vi "Configure VIs for Execution.vi"   [LabVIEW 2016, in "Memory.lvlib"]
uses:
  Memory.lvlib
types:
  T1 = enum32{"invalid VI type", "Standard VI", "Control VI", "Global VI", "Polymorphic VI", "Configuration VI", "SubSystem", "Facade VI", "Method VI", "Statechart Diagram VI"}
  T2 = enum16{"Share clones between instances", "Preallocate clone for each instance"}
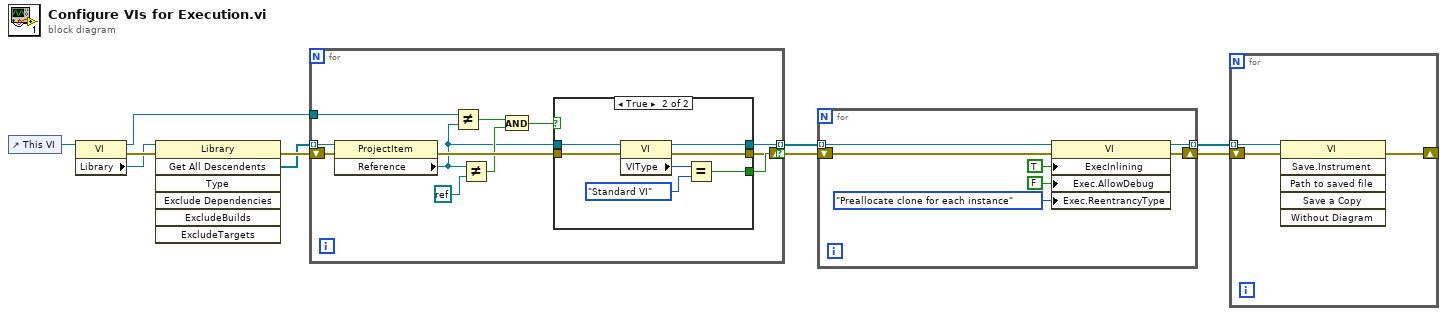
[diagram p0: block diagram]
diagram:
  n1 = control-ref of="This VI"() -> (w10:refnum<vi>)
  n2 = property class="VI"(reference=w10) -> (reference out=w8:refnum<vi>, error out=w3:errorcluster, "Library"=w1:refnum<vi>)  [unwired: 1 in]
  n3 = invoke class="Library" method="Get All Descendents"(reference=w1, error in=w3) -> (error out=w4:errorcluster, "All Descendents"=w2:refnum<vi>[])  [unwired: 5 in, 5 out]
  n4 = for {
    tunnel: w2 -> [w22] mode=indexing
    tunnel: [w21] -> w9 mode=indexing if=w20
    tunnel: w8 -> [w18]
    shift-right: [w16] -> w7
    shift-left: w4 -> [w15]
    n5 = property class="ProjectItem"(reference=w22, error in=w15) -> (error out=w14:errorcluster, "Reference"=w11:refnum<vi>)  [unwired: 1 out]
    n6 = Not Equal?(x=w18, y=w11) -> (x != y?=w17:bool)
    n7 = Not Equal?(x=w11, y=refnum<k0> refnum) -> (x != y?=w13:bool)
    n8 = And(x=w17, y=w13) -> (x .and. y?=w12:bool)
    n9 = case shown="True" w12 {
      selector: w12 -> [w24 _]
      tunnel: [w25 w31] -> w21
      tunnel: [w24 w30] -> w20
      tunnel: w11 -> [w25 w28]
      tunnel: [w23 w27] -> w16
      tunnel: w14 -> [w23 w26]
      frame False {
      }
      frame True {
        n10 = property class="VI"(reference=w28, error in=w26) -> (reference out=w31:refnum<vi>, error out=w27:errorcluster, "VIType"=w32:T1)
        n11 = Equal?(x=w32, y=T1."Standard VI" ("VI Type")) -> (x = y?=w30:bool)
      }
    }
  }
  n12 = for {
    tunnel: w9 -> [w39] mode=indexing
    tunnel: [w37] -> w6 mode=indexing
    shift-right: [w36] -> w5
    shift-left: w7 -> [w38]
    n13 = property class="VI"(reference=w39, error in=w38, "ExecInlining"=TRUE ("Execution:Inline SubVI"), "Exec.AllowDebug"=FALSE ("Execution:Allow Debugging"), "Exec.ReentrancyType"=T2."Preallocate clone for each instance" ("Execution:Reentrancy Type")) -> (reference out=w37:refnum<vi>, error out=w36:errorcluster)
  }
  n14 = for {
    tunnel: w6 -> [w41] mode=indexing
    shift-right: [w40] -> _
    shift-left: w5 -> [w42]
    n15 = invoke class="VI" method="Save.Instrument"(reference=w41, error in=w42) -> (error out=w40:errorcluster)  [unwired: 4 in, 5 out]
  }
